vi "Arrays_Bool Set Size.vi"(3 "Array":bool[](array[boolean]), 4 "Size":i32) -> (5 "Array Out":bool[](array[boolean]))   [LabVIEW 2015]
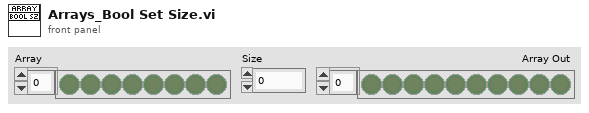
[diagram p1: front panel]
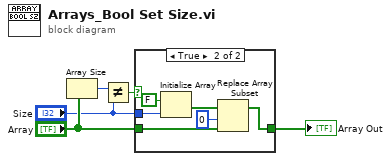
[diagram p0: block diagram]
diagram:
  n1 = Array Size(array="Array") -> (size(s)=w3:i32)
  n2 = Not Equal?(x=w3, y="Size") -> (x != y?=w1:bool)
  n3 = case shown="True" w1 {
    tunnel: [w6 w12] -> w5
    tunnel: "Size" -> [_ w8]
    tunnel: "Array" -> [w6 w7]
    frame False {
    }
    frame True {
      n4 = Initialize Array(FALSE, w8) -> (w10:bool[])
      n5 = Replace Array Subset(array=w10, new element=w7, index=0) -> (w12:bool[])
    }
  }
  "Array Out" <- w5
